vi "start.vi"(8 "error in (no error)":errorcluster, 10 "soundOnly?":bool, 11 "HWController in":refnum<class "HWController.lvclass">) -> (0 "error out":errorcluster, 2 "started?":bool, 3 "HWController out":refnum<class "HWController.lvclass">)   [LabVIEW 2009, in "Hardware.lvlib" / "HWControllers.lvlib" / "HWController.lvclass"]
uses:
  HWController.lvclass
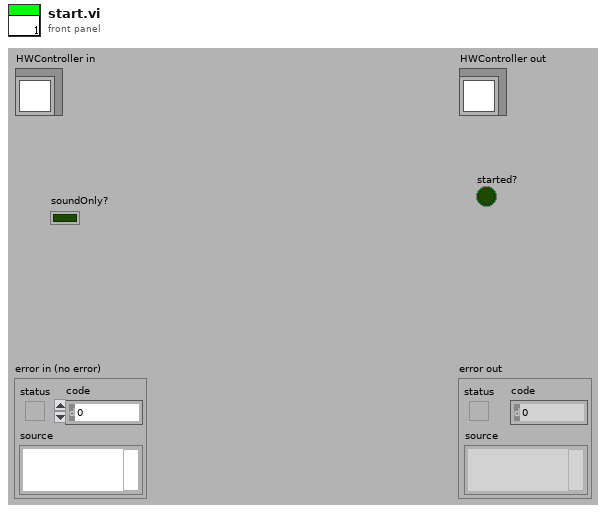
[diagram p1: front panel]
types:
  T1 = enum16{"Ready", "Compiling", "Configured", "Running", "Stopping", "Unresolved Error"}
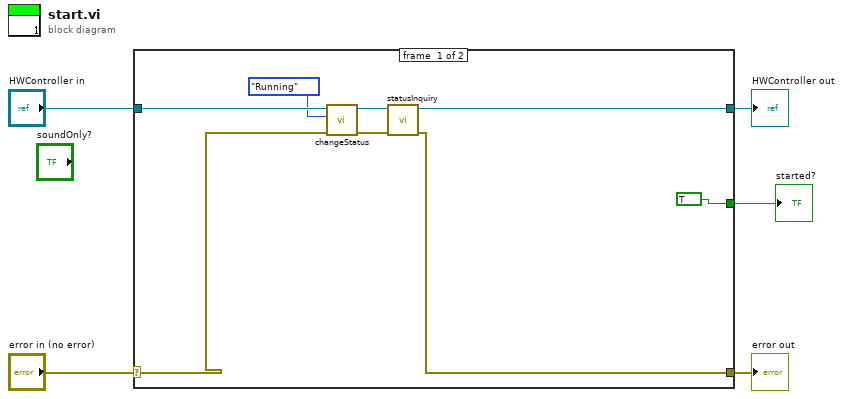
[diagram p0: block diagram]
diagram:
  n1 = case shown="No Error" "error in (no error)" {
    selector: "error in (no error)" -> [w9 w15]
    tunnel: [w8 w15] -> w4
    tunnel: [w11 w14] -> w2
    tunnel: "HWController in" -> [w10 w14]
    tunnel: [TRUE _] -> w1
    frame #0 {
      n2 = call "changeStatus.vi"("error in (no error)"=w9, "status"=T1."Running", "HWController in"=w10) -> ("error out"=w13:errorcluster, "HWController out"=w12:refnum<class "HWController.lvclass">)  [unwired: 7 in]
      n3 = call-dynamic "statusInquiry.vi"("error in (no error)"=w13, "HWController in"=w12) -> ("error out"=w8:errorcluster, "HWController out"=w11:refnum<class "HWController.lvclass">)  [unwired: 8 in]
    }
    frame #1 {
    }
  }
  "error out" <- w4
  "HWController out" <- w2
  "started?" <- w1
